vi "Vector Circle Intersection.vi"(8 "error in (no error)":errorcluster, 9 "Circle Center":cluster{"x":dbl, "y":dbl}={"x"=2.0, "y"=0.0}, 10 "Vector Bearing":dbl=0.1, 11 "Circle Radius":dbl=0.1) -> (0 "error out":errorcluster, 2 "Intersection?":bool, 3 "Points of Intersection":cluster{dbl, dbl}[](array[cluster]))   [LabVIEW 2011]
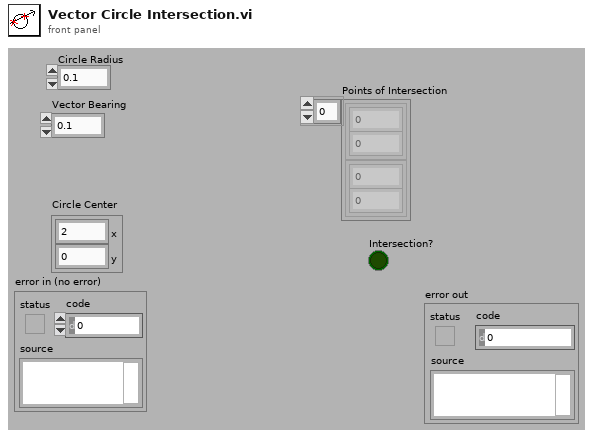
[diagram p1: front panel]
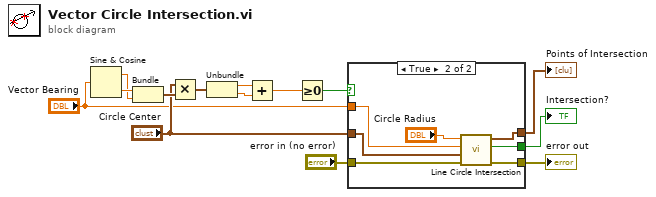
[diagram p0: block diagram]
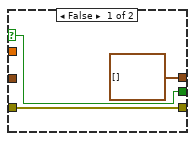
[diagram p2: hidden frame]
diagram:
  n1 = Sine & Cosine(0:"Vector Bearing") -> (1:w12:dbl, 2:w13:dbl)
  n2 = Bundle(w13, w12) -> (w11:cluster{dbl, dbl})  [unwired: 1 in]
  n3 = Multiply(x="Circle Center", y=w11) -> (x*y=w9:cluster{dbl, dbl})
  n4 = Unbundle(w9) -> (w8:dbl, w7:dbl)
  n5 = Add(x=w8, y=w7) -> (x+y=w6:dbl)
  n6 = Greater Or Equal To 0?(x=w6) -> (x >= 0?=w5:bool)
  n7 = case shown="True" w5 {
    selector: w5 -> [w15 _]
    tunnel: [cluster{dbl, dbl}[] [] ("Points of Intersection") w23] -> w14
    tunnel: "Vector Bearing" -> [_ w22]
    tunnel: "Circle Center" -> [_ w21]
    tunnel: "error in (no error)" -> [w16 w20]
    tunnel: [w16 w19] -> w3
    tunnel: [w15 w18] -> w2
    frame False {
    }
    frame True {
      n8 = call "Line Circle Intersection.vi"("error in (no error)"=w20, "Circle Center"=w21, "Line's Angle (rads)"=w22, "Circle Radius"="Circle Radius") -> ("error out"=w19:errorcluster, "Intersection?"=w18:bool, "Points of Intersection"=w23:cluster{dbl, dbl}[])  [unwired: 5 in]
    }
  }
  "Points of Intersection" <- w14
  "error out" <- w3
  "Intersection?" <- w2
